vi "Scale Channel Data.vi"(8 "error in (no error)":errorcluster, 9 "Channel Index":i32=-1, 10 "Data":dbl[](array[numeric]), 11 "Scaling in":refnum<class "Scaling.lvclass">) -> (0 "error out":errorcluster, 2 "Scaled Data":dbl[](array[numeric]), 3 "Scaling out":refnum<class "Scaling.lvclass">)   [LabVIEW 2020, in "VolatusData.lvlib" / "Scaling.lvclass"]
uses:
  Scaling.lvclass
  Scaling.lvclass/Scaling.ctl
  Polynomial Remove Trailing Zeros.vi
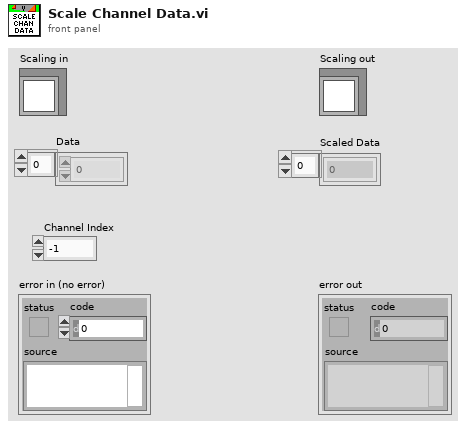
[diagram p1: front panel]
types:
  T1 = typedef "VolatusConfig.lvlib/Scale Type.ctl" = enum16{"None", "Sensor", "Polynomial", "Threshold", "Invert Bool"}
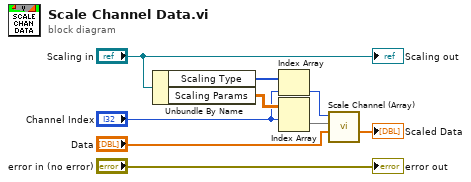
[diagram p0: block diagram]
diagram:
  n1 = Unbundle By Name("Scaling in") -> ("Scaling Type"=w7:T1[], "Scaling Params"=w6:dbl[][])
  n2 = Index Array(array=w7, index="Channel Index") -> (element=w4:T1)
  n3 = Index Array(array=w6, index (row)="Channel Index") -> (element=w3:dbl[])  [unwired: 1 in]
  n4 = call "Scale Channel (Array).vi"("Data"="Data", "Scaling Params"=w3, "Scaling Type"=w4) -> ("Scaled Data"=→"Scaled Data":dbl[])  [unwired: 8 in]
  "error out" <- "error in (no error)"
  "Scaling out" <- "Scaling in"
